vi "CMI ADS127L21 - Read Record Data.vi"(8 "error in (no error)":errorcluster, 11 "session in":T1 {"channels"."Channel" min=1 max=8 step=1}) -> (0 "error out":errorcluster, 1 "done?":bool, 2 "Raw Sample Data (column per channel)":i32[][](array[numeric]), 3 "session out":T1 {"channels"."Channel" min=1 max=8 step=1}, 4 "sample offset":i32, 5 "FIFO usage [%]":dbl, 6 "sample count":i32)   [LabVIEW 2020]
doc: "Read chunk of record data."
uses:
  CMI ADS127L21 - Session.ctl
  CMI ADS127L21 - Record Channel.ctl
  CMI ADS127L21 - Input Range.ctl
  CMI ADS127L21 - Input Mode.ctl
  CMI ADS127L21 - Input Impedance.ctl
  CMI ADS127L21 - EXTOUT Mode.ctl
  CMI ADS127L21 - EXTOUT Polarity.ctl
  <vilib>/Instr/_visa.llb/VISA Flush IO Buffer Mask.ctl
  <vilib>/Utility/error.llb/Error Cluster From Error Code.vi
  <vilib>/ErrorRing/Error Ring.xnode
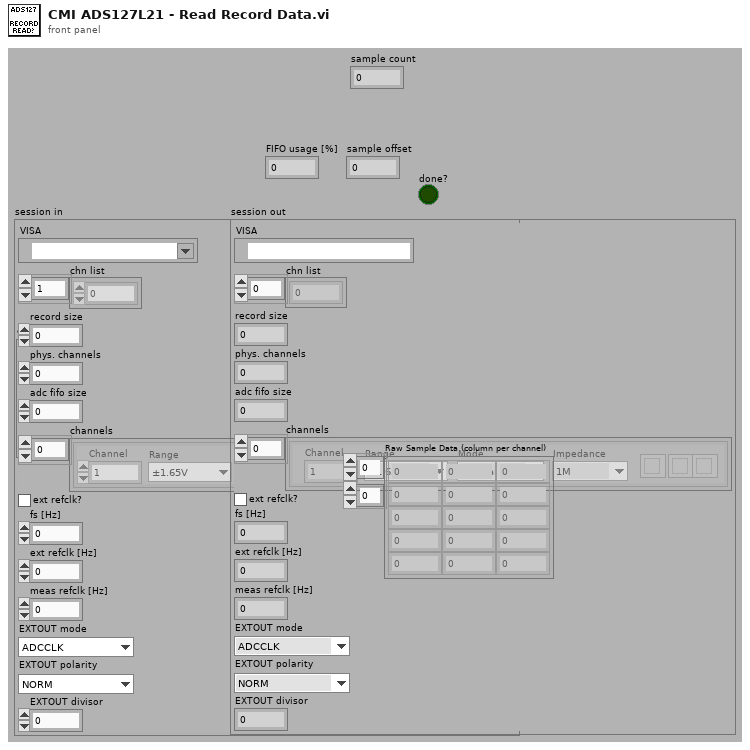
[diagram p1: front panel]
types:
  T1 = typedef "CMI ADS127L21 - Session.ctl" = cluster{"VISA":refnum<visa-resource-name>, "chn list":i32[], "record size":i32, "phys. channels":i32, "adc fifo size":i32, "channels":T2[], "ext refclk?":bool, "fs [Hz]":dbl, "ext refclk [Hz]":dbl, "meas refclk [Hz]":dbl, "EXTOUT mode":T6, "EXTOUT polarity":T7, "EXTOUT divisor":i32}
  T2 = typedef "CMI ADS127L21 - Record Channel.ctl" = cluster{"Range":T3, "Channel":i32, "Mode":T4, "Impedance":T5, "btn clr":bool, "btn up":bool, "btn down":bool}
  T3 = typedef "CMI ADS127L21 - Input Range.ctl" = enum16{"±1.65V", "±2V"}
  T4 = typedef "CMI ADS127L21 - Input Mode.ctl" = enum16{"Normal", "Inverted", "GND"}
  T5 = typedef "CMI ADS127L21 - Input Impedance.ctl" = enum16{"1M", "1k5"}
  T6 = typedef "CMI ADS127L21 - EXTOUT Mode.ctl" = enum16{"ADCCLK", "REFCLK", "SMPLCLK", "FIRST"}
  T7 = typedef "CMI ADS127L21 - EXTOUT Polarity.ctl" = enum16{"NORM", "INV"}
  T8 = enum16{"big-endian, network order", "native, host order", "little-endian"}
  T9 = typedef "VISA Flush IO Buffer Mask.ctl" = u16
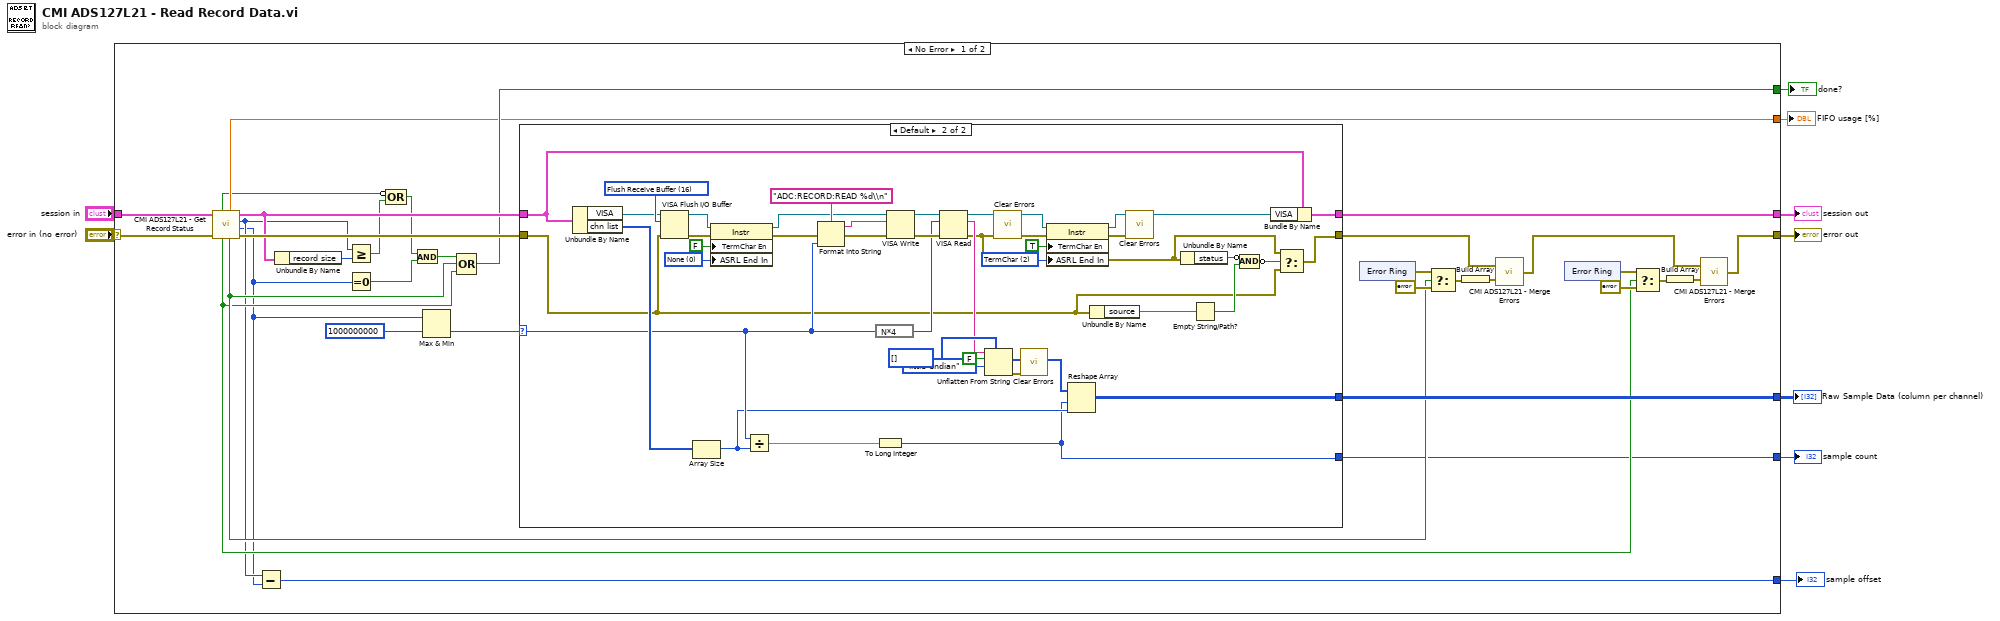
[diagram p0: block diagram]
diagram:
  n1 = case shown="No Error" "error in (no error)" {
    selector: "error in (no error)" -> [w40 w97]
    tunnel: "session in" -> [w37 w96]
    tunnel: [w42 w96] -> w8
    tunnel: [w24 w97] -> w7
    tunnel: [w41 _] -> w5
    tunnel: [w22 _] -> w4
    tunnel: [w17 _] -> w3
    tunnel: [w14 _] -> w2
    tunnel: [w13 _] -> w1
    frame No Error {
      n2 = call "CMI ADS127L21 - Get Record Status.vi"("error in (no error)"=w40, "session in"=w37) -> ("error out"=w39:errorcluster, "samples to read"=w15:i32, "samples acquired"=w16:i32, "session out"=w38:T1, "FIFO overflow?"=w21:bool, "FIFO usage [%]"=w17:dbl, "sampling error"=w20:bool, "record running?"=w10:bool)  [unwired: 2 in]
      n3 = Subtract(x=w16, y=w15) -> (x-y=w14:i32)
      n4 = Unbundle By Name(w38) -> ("record size"=w36:i32)
      n5 = Greater Or Equal?(x=w16, y=w36) -> (x >= y?=w11:bool)
      n6 = Equal To 0?(x=w15) -> (x = 0?=w35:bool)
      n7 = Compound Arithmetic op=OR(invert w10, w11) -> (w12:bool)
      n8 = Compound Arithmetic op=AND(w12, w35) -> (w23:bool)
      n9 = Max & Min(x=w15, y=1000000000) -> (min(x,y)=w19:i32)  [unwired: 1 out]
      n10 = Compound Arithmetic op=OR(w23, w21, w20) -> (w22:bool)
      n11 = case shown="Default" w19 {
        selector: w19 -> [_ w68]
        tunnel: [w53 w95] -> w42
        tunnel: w38 -> [w53 w94]
        tunnel: w39 -> [w54 w57]
        tunnel: [w54 w80] -> w30
        tunnel: [_ w76] -> w41
        tunnel: [_ w55] -> w13
        frame 0 {
        }
        frame Default {
          w60 = u16 2 items=["None", "Last Bit", "TermChar"] ("Serial Settings:End Mode for Reads")
          w61 = u16 0 items=["None", "Last Bit", "TermChar"] ("Serial Settings:End Mode for Reads")
          w92 = T9 16 items=["Flush Receive Buffer"=16, "Write Transmit Buffer to Device"=32, "Flush Receive Buffer (No I/O)"=64, "Flush Transmit Buffer"=128] ("Mask")
          n12 = Unbundle By Name(w94) -> ("VISA"=w90:refnum<visa-resource-name>, "chn list"=w78:i32[])
          n13 = VISA Flush I/O Buffer(VISA resource name=w90, mask (16)=w92, error in (no error)=w57) -> (VISA resource name out=w66:refnum<visa-resource-name>, error out=w91:errorcluster)
          n14 = Array Size(array=w78) -> (size(s)=w56:i32)
          n15 = property class="Instr"(reference=w66, error in=w91, "TermChar En"=FALSE ("Message Based Settings:Termination Character Enable"), "ASRL End In"=w61) -> (reference out=w65:refnum<visa-resource-name>, error out=w93:errorcluster)
          n16 = Divide(x=w68, y=w56) -> (x/y=w77:dbl)
          n17 = Format Into String(format string="ADC:RECORD:READ %d\\n", error in=w93, w68) -> (resulting string=w67:string, error out=w59:errorcluster)  [unwired: 1 in]
          n18 = expression code="N*4"(w68) -> (w79:i32)
          n19 = To Long Integer(number=w77) -> (32bit integer=w55:i32)
          n20 = VISA Write(VISA resource name=w65, write buffer=w67, error in (no error)=w59) -> (VISA resource name out=w88:refnum<visa-resource-name>, error out=w89:errorcluster)  [unwired: 1 out]
          n21 = VISA Read(VISA resource name=w88, byte count=w79, error in (no error)=w89) -> (VISA resource name out=w87:refnum<visa-resource-name>, read buffer=w62:string, error out=w58:errorcluster)  [unwired: 1 out]
          n22 = Unflatten From String(type=i32[] [], binary string=w62, data includes array or string size? (T)=FALSE, byte order (0:big-endian, network order)=T8."little-endian") -> (value=w73:i32[], error out=w72:errorcluster)  [unwired: 1 in, 1 out]
          n23 = call <vilib>:"Clear Errors.vi"("error in (no error)"=w58) -> ("error out"=w75:errorcluster)  [unwired: 5 in, 1 out]
          n24 = call <vilib>:"Clear Errors.vi"("error in (no error)"=w72) -> ()  [unwired: 5 in, 2 out]
          n25 = property class="Instr"(reference=w87, error in=w75, "TermChar En"=TRUE ("Message Based Settings:Termination Character Enable"), "ASRL End In"=w60) -> (reference out=w86:refnum<visa-resource-name>, error out=w81:errorcluster)
          n26 = Reshape Array(w73, w55, w56) -> (w76:i32[][])
          n27 = Unbundle By Name(w57) -> ("source"=w85:string)
          n28 = call <vilib>:"Clear Errors.vi"("error in (no error)"=w81) -> ()  [unwired: 5 in, 2 out]
          n29 = Unbundle By Name(w58) -> ("status"=w84:bool)
          n30 = Empty String/Path?(string/path=w85) -> (empty?=w83:bool)
          n31 = Compound Arithmetic op=AND(invert w84, w83) -> (invert w82:bool)
          n32 = Bundle By Name(cluster=w94, "VISA"=w86) -> (w95:T1)
          n33 = Select(t=w58, s=w82, f=w57) -> (s? t:f=w80:errorcluster)
        }
      }
      n34 = xnode "Error Ring"() -> ("error out"=w34:errorcluster)
      n35 = Select(t=w34, s=w21, f=errorcluster {"status"=FALSE, "code"=0, "source"=""}) -> (s? t:f=w33:errorcluster)
      n36 = Build Array(w33) -> (w32:errorcluster[])
      n37 = call "CMI ADS127L21 - Merge Errors.vi"("errors in"=w32, "error in (no error)"=w30) -> ("error out"=w25:errorcluster)
      n38 = xnode "Error Ring"() -> ("error out"=w26:errorcluster)
      n39 = Select(t=w26, s=w20, f=errorcluster {"status"=FALSE, "code"=0, "source"=""}) -> (s? t:f=w27:errorcluster)
      n40 = Build Array(w27) -> (w28:errorcluster[])
      n41 = call "CMI ADS127L21 - Merge Errors.vi"("errors in"=w28, "error in (no error)"=w25) -> ("error out"=w24:errorcluster)
    }
    frame Error {
    }
  }
  "error out" <- w7
  "session out" <- w8
  "Raw Sample Data (column per channel)" <- w5
  "done?" <- w4
  "FIFO usage [%]" <- w3
  "sample offset" <- w2
  "sample count" <- w1
